vi "AuMT8852B Notify When Operation Complete.vi"(8 "error in (no error)":errorcluster, 11 "VISA session":refnum<visa-resource-name>) -> (0 "error out":errorcluster, 2 "error code":i32, 3 "VISA session out":refnum<visa-resource-name>)   [LabVIEW 2017]
doc: "Anritsu MT8852B Bluetooth Tester\n\nTells the instrument to send a Service Request (SRQ) when a pending operation completes."
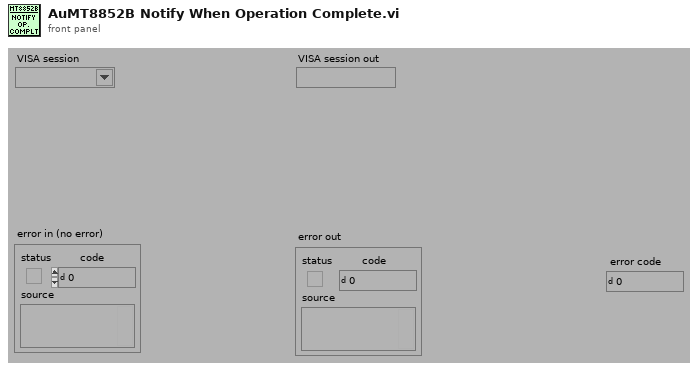
[diagram p1: front panel]
types:
  T1 = enum16{"Simulate", "Range check", "Cache", "Query instrument status"}
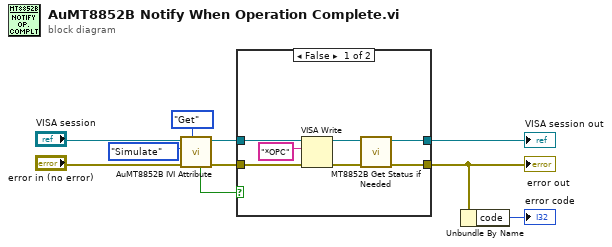
[diagram p0: block diagram]
diagram:
  n1 = call <instrlib>:"AuMT8852B IVI Attribute.vi"("Set/Get (Set)"=enum16{"Set", "Get"}."Get", "error in (no error)"="error in (no error)", "Flag (Simulate)"=T1."Simulate", "VISA session"="VISA session") -> ("error out"=w6:errorcluster, "VISA session out"=w7:refnum<visa-resource-name>, "Value out"=w3:bool)  [unwired: 5 in]
  n2 = case shown="False" w3 {
    tunnel: [w17 w18] -> w10
    tunnel: [w16 w19] -> w1
    tunnel: w7 -> [w15 w18]
    tunnel: w6 -> [w14 w19]
    frame False {
      n3 = VISA Write(VISA resource name=w15, write buffer="*OPC" ("write buffer (\"\")"), error in (no error)=w14) -> (VISA resource name out=w13:refnum<visa-resource-name>, error out=w12:errorcluster)  [unwired: 1 out]
      n4 = call <instrlib>:"MT8852B Get Status if Needed.vi"("error in (no error)"=w12, "VISA session"=w13) -> ("error out"=w16:errorcluster, "VISA session out"=w17:refnum<visa-resource-name>)  [unwired: 8 in]
    }
    frame True {
    }
  }
  "VISA session out" <- w10
  "error out" <- w1
  n5 = Unbundle By Name(w1) -> ("code"=→"error code":i32)
